vi "Send TCP Command.vi"(7 "Action":T1, 8 "error in (no error)":errorcluster, 10 "Custom Message":string, 11 "Telnet V2 in":refnum<class "UDP.lvclass">) -> (0 "error out":errorcluster, 3 "Telnet V2 out":refnum<class "UDP.lvclass">)   [LabVIEW 2018]
uses:
  Controls/enum_Telnet_Actions.ctl
  UDP.lvclass
  PPLs/LiDAR/Parent/LiDAR.lvlibp/Controls/enm_Actions_for_LiDAR.ctl
  PPLs/LiDAR/Parent/LiDAR.lvlibp/LiDAR.lvclass
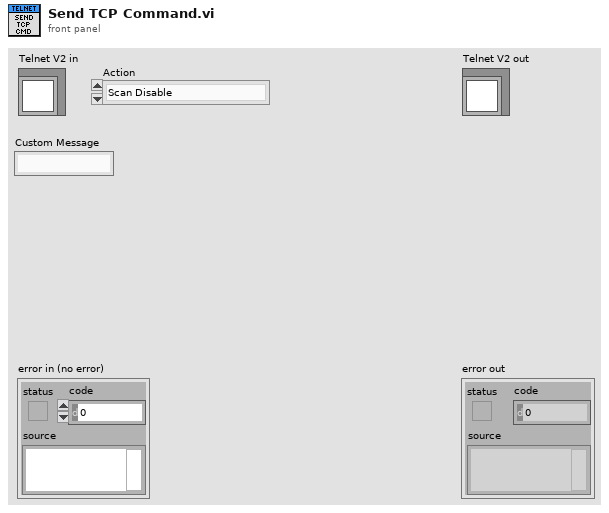
[diagram p1: front panel]
types:
  T1 = typedef "LiDAR.lvlibp/LiDAR.lvclass/enm_Actions_for_LiDAR.ctl" = enum16{"Scan Disable", "Scan Enable", "Standby", "Active", "Change EL Scan", "Change AZ Scan", "Change Algo", "Custom"}
  T2 = typedef "UDP.lvlib/UDP.lvclass/enum_Telnet_Actions.ctl" = enum16{"Scan Enable", "Scan Disable", "Active", "Standby", "Change EL Scan", "Change AZ Scan", "Set Data Algo", "Debug System", "Debug Laser", "Exit"}
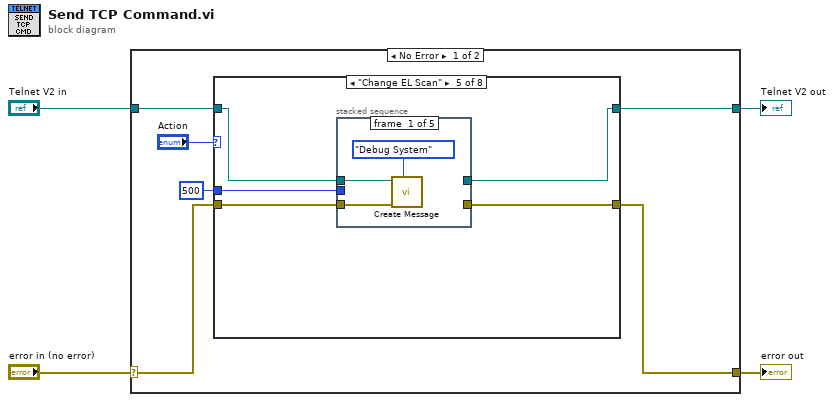
[diagram p0: block diagram]
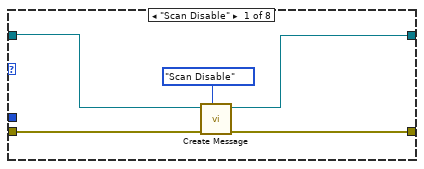
[diagram p2: hidden frame]
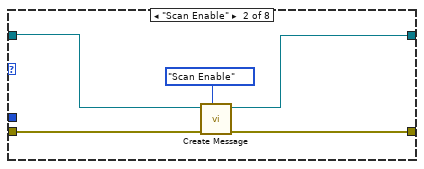
[diagram p3: hidden frame]
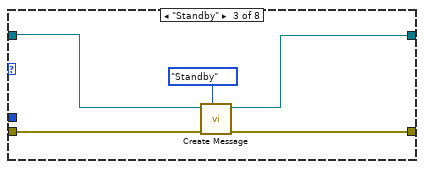
[diagram p4: hidden frame]
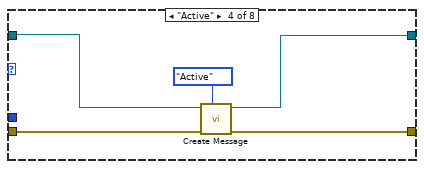
[diagram p5: hidden frame]
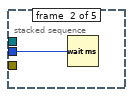
[diagram p6: hidden frame]
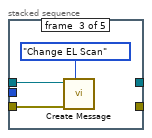
[diagram p7: hidden frame]
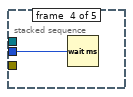
[diagram p8: hidden frame]
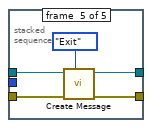
[diagram p9: hidden frame]
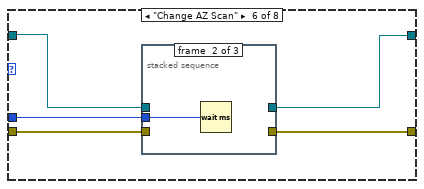
[diagram p10: hidden frame]
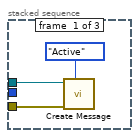
[diagram p11: hidden frame]
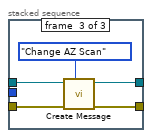
[diagram p12: hidden frame]
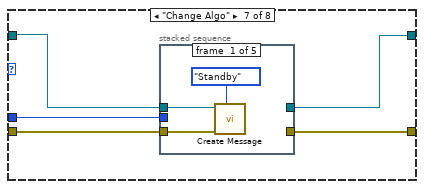
[diagram p13: hidden frame]
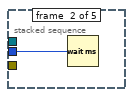
[diagram p14: hidden frame]
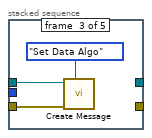
[diagram p15: hidden frame]
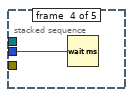
[diagram p16: hidden frame]
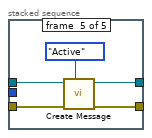
[diagram p17: hidden frame]
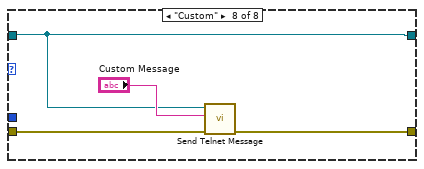
[diagram p18: hidden frame]
diagram:
  n1 = case shown="No Error" "error in (no error)" {
    selector: "error in (no error)" -> [w8 w86]
    tunnel: [w7 w86] -> w3
    tunnel: [w6 w85] -> w1
    tunnel: "Telnet V2 in" -> [w9 w85]
    frame No Error {
      n2 = case shown="\"Change EL Scan\"" "Action" {
        tunnel: w9 -> [w14 w19 w24 w29 w34 w50 w65 w81]
        tunnel: w8 -> [w12 w17 w21 w27 w35 w53 w67 w83]
        tunnel: [w11 w16 w22 w26 w33 w52 w66 w82] -> w7
        tunnel: [w13 w18 w23 w28 w32 w51 w64 w81] -> w6
        tunnel: u32 500 ("milliseconds to wait") -> [_ _ _ _ w31 w49 w63 _]
        frame "Scan Disable" {
          n3 = call "Create Message.vi"("Action"=enum_Telnet_Actions."Scan Disable", "error in (no error)"=w12, "Telnet V2 in"=w14) -> ("error out"=w11:errorcluster, "Telnet V2 Out"=w13:refnum<class "UDP.lvclass">)  [unwired: 7 in]
        }
        frame "Scan Enable" {
          n4 = call "Create Message.vi"("Action"=enum_Telnet_Actions."Scan Enable", "error in (no error)"=w17, "Telnet V2 in"=w19) -> ("error out"=w16:errorcluster, "Telnet V2 Out"=w18:refnum<class "UDP.lvclass">)  [unwired: 7 in]
        }
        frame "Standby" {
          n5 = call "Create Message.vi"("Action"=enum_Telnet_Actions."Standby", "error in (no error)"=w21, "Telnet V2 in"=w24) -> ("error out"=w22:errorcluster, "Telnet V2 Out"=w23:refnum<class "UDP.lvclass">)  [unwired: 7 in]
        }
        frame "Active" {
          n6 = call "Create Message.vi"("Action"=enum_Telnet_Actions."Active", "error in (no error)"=w27, "Telnet V2 in"=w29) -> ("error out"=w26:errorcluster, "Telnet V2 Out"=w28:refnum<class "UDP.lvclass">)  [unwired: 7 in]
        }
        frame "Change EL Scan" {
          n7 = stacked-sequence {
            tunnel: w34 -> [w37 _ w41 _ w47]
            tunnel: w35 -> [w36 _ w40 _ w46]
            tunnel: [_ _ _ _ w45] -> w33
            tunnel: [_ _ _ _ w44] -> w32
            tunnel: w31 -> [_ w39 _ w43 _]
            frame #0 {
              n8 = call "Create Message.vi"("Action"=enum_Telnet_Actions."Debug System", "error in (no error)"=w36, "Telnet V2 in"=w37) -> ()  [unwired: 7 in, 2 out]
            }
            frame #1 {
              n9 = Wait (ms)(milliseconds to wait=w39) -> ()  [unwired: 1 out]
            }
            frame #2 {
              n10 = call "Create Message.vi"("Action"=enum_Telnet_Actions."Change EL Scan", "error in (no error)"=w40, "Telnet V2 in"=w41) -> ()  [unwired: 7 in, 2 out]
            }
            frame #3 {
              n11 = Wait (ms)(milliseconds to wait=w43) -> ()  [unwired: 1 out]
            }
            frame #4 {
              n12 = call "Create Message.vi"("Action"=enum_Telnet_Actions."Exit", "error in (no error)"=w46, "Telnet V2 in"=w47) -> ("error out"=w45:errorcluster, "Telnet V2 Out"=w44:refnum<class "UDP.lvclass">)  [unwired: 7 in]
            }
          }
        }
        frame "Change AZ Scan" {
          n13 = stacked-sequence {
            tunnel: w50 -> [w55 _ w61]
            tunnel: w53 -> [w54 _ w60]
            tunnel: [_ _ w59] -> w52
            tunnel: [_ _ w58] -> w51
            tunnel: w49 -> [_ w57 _]
            frame #0 {
              n14 = call "Create Message.vi"("Action"=enum_Telnet_Actions."Active", "error in (no error)"=w54, "Telnet V2 in"=w55) -> ()  [unwired: 7 in, 2 out]
            }
            frame #1 {
              n15 = Wait (ms)(milliseconds to wait=w57) -> ()  [unwired: 1 out]
            }
            frame #2 {
              n16 = call "Create Message.vi"("Action"=enum_Telnet_Actions."Change AZ Scan", "error in (no error)"=w60, "Telnet V2 in"=w61) -> ("error out"=w59:errorcluster, "Telnet V2 Out"=w58:refnum<class "UDP.lvclass">)  [unwired: 7 in]
            }
          }
        }
        frame "Change Algo" {
          n17 = stacked-sequence {
            tunnel: w65 -> [w69 _ w73 _ w79]
            tunnel: w67 -> [w68 _ w72 _ w78]
            tunnel: [_ _ _ _ w77] -> w66
            tunnel: [_ _ _ _ w76] -> w64
            tunnel: w63 -> [_ w71 _ w75 _]
            frame #0 {
              n18 = call "Create Message.vi"("Action"=enum_Telnet_Actions."Standby", "error in (no error)"=w68, "Telnet V2 in"=w69) -> ()  [unwired: 7 in, 2 out]
            }
            frame #1 {
              n19 = Wait (ms)(milliseconds to wait=w71) -> ()  [unwired: 1 out]
            }
            frame #2 {
              n20 = call "Create Message.vi"("Action"=enum_Telnet_Actions."Set Data Algo", "error in (no error)"=w72, "Telnet V2 in"=w73) -> ()  [unwired: 7 in, 2 out]
            }
            frame #3 {
              n21 = Wait (ms)(milliseconds to wait=w75) -> ()  [unwired: 1 out]
            }
            frame #4 {
              n22 = call "Create Message.vi"("Action"=enum_Telnet_Actions."Active", "error in (no error)"=w78, "Telnet V2 in"=w79) -> ("error out"=w77:errorcluster, "Telnet V2 Out"=w76:refnum<class "UDP.lvclass">)  [unwired: 7 in]
            }
          }
        }
        frame "Custom" {
          n23 = call "Send Telnet Message.vi"("error in"=w83, "Message In"="Custom Message", "Telnet V2 in"=w81) -> ("error out"=w82:errorcluster)  [unwired: 8 in]
        }
      }
    }
    frame Error {
    }
  }
  "error out" <- w3
  "Telnet V2 out" <- w1
